vi "EngineCommandTest.vi"() -> ()   [LabVIEW 2020]
uses:
  Command.ctl
  393a57cb-fd34-42c5-83ef-d732c095d0a3.vi
  <vilib>/Instr/_visa.llb/VISA Configure Serial Port (Instr).vi
  PicoG-Core.lvlib
panel:
  out "error out":errorcluster
  out "read buffer":string
  in  "Port":refnum<visa-resource-name>
  in  "Command":T1
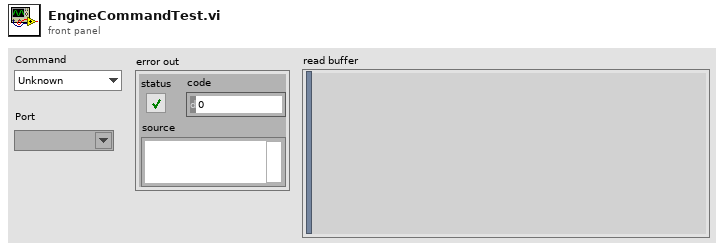
[diagram p1: front panel]
types:
  T1 = typedef "PicoG-Core.lvlib/Command.ctl" = enum8{"Unknown", "Version", "Platform", "Board", "Serial", "Alias", "IsExec", "Reset", "Abort", "RunMain", "SkipStartup"}
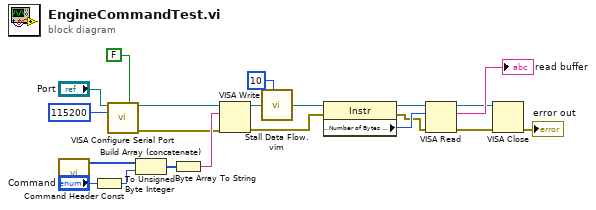
[diagram p0: block diagram]
diagram:
  n1 = call "Command Header Const.vi"() -> ("Command Header"=w20:u8[])  [unwired: 11 in]
  n2 = To Unsigned Byte Integer(number="Command") -> (unsigned 8bit integer=w19:u8)
  n3 = call-poly "VISA Configure Serial Port"("VISA resource name"="Port", "Enable Termination\nChar (T)"=FALSE ("Enable Termination\nChar (T)"), "baud rate (9600)"=u32 115200) -> ("VISA resource name out"=w14:refnum<visa-resource-name>, "error out"=w2:errorcluster)  [unwired: 11 in]
  n4 = Build Array (concatenate)(w20, w19) -> (w18:u8[])
  n5 = Byte Array To String(unsigned byte array=w18) -> (string=w13:string)
  n6 = VISA Write(VISA resource name=w14, write buffer=w13, error in (no error)=w2) -> (VISA resource name out=w12:refnum<visa-resource-name>, error out=w6:errorcluster)  [unwired: 1 out]
  n7 = call "Stall Data Flow.vim"("value in"=w12, "milliseconds to wait"=u32 10) -> ("value out"=w10:refnum<visa-resource-name>)  [unwired: 1 out]
  n8 = property class="Instr"(reference=w10, error in=w6) -> (reference out=w9:refnum<visa-resource-name>, error out=w7:errorcluster, "Serial Settings:Number of Bytes at Serial Port"=w8:u32)
  n9 = VISA Read(VISA resource name=w9, byte count=w8, error in (no error)=w7) -> (VISA resource name out=w4:refnum<visa-resource-name>, read buffer=→"read buffer":string, error out=w3:errorcluster)  [unwired: 1 out]
  n10 = VISA Close(VISA resource name=w4, error in (no error)=w3) -> (error out=→"error out":errorcluster)
